vi "Connected.vi"(8 "error in (no error)":errorcluster, 10 "Connected Argument":T1) -> (0 "error out":errorcluster)   [LabVIEW 2015, in "Tool Module.lvlib"]
doc: "Returns status of connecting/disconnecting from the tool.\n_____\nCreated using Delacor QMH Event Scripter 2.1.0.3."
uses:
  Tool Module.lvlib
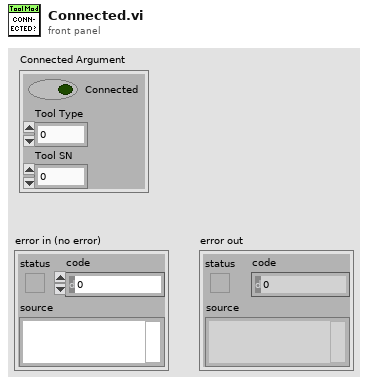
[diagram p1: front panel]
types:
  T1 = cluster{"Connected":bool, "Tool Type":u16, "Tool SN":u16}
  T2 = typedef "Tool Module.lvlib/Broadcast Events--cluster.ctl" = cluster{"Module Did Init":refnum<user-event>, "Status Updated":refnum<user-event>, "Error Reported":refnum<user-event>, "Module Did Stop":refnum<user-event>, "Update Module Execution Status":refnum<user-event>, "Send Status":refnum<user-event>, "Trigger":refnum<user-event>, "Connected":refnum<user-event>, "Read from File Rtn":refnum<user-event>, "Device Temperature":refnum<user-event>}
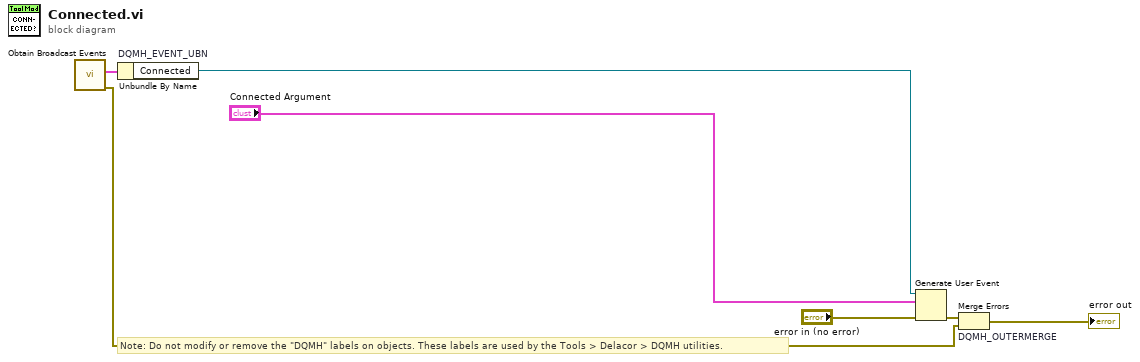
[diagram p0: block diagram]
diagram:
  # "Note: Do not modify or remove the \"DQMH\" labels on objects. These labels are used by the Tools > Delacor > DQMH utilities."
  n1 = call "Obtain Broadcast Events.vi"() -> ("error out"=w3:errorcluster, "Tool Module Broadcast Events"=w2:T2)  [unwired: 10 in]
  n2 = Unbundle By Name "DQMH_EVENT_UBN"(w2) -> ("Connected"=w5:refnum<user-event>)
  n3 = Generate User Event(user event=w5, event data cluster="Connected Argument", error in="error in (no error)") -> (error out=w4:errorcluster)  [unwired: 1 in, 1 out]
  n4 = Merge Errors "DQMH_OUTERMERGE"(w4, w3) -> (→"error out":errorcluster)
